vi "Draw Caster Wheel Forward Velocity.vi"(6 "wheel state":T1, 7 "picture info":T3={"picture size"={"Width"=500, "Height"=500}, "pixels per unit"=10.0}, 8 "error in (no error)":errorcluster, 9 "draw wheel options":T2={"global wheel position"={"x"=0.0, "y"=0.0}, "wheel frame angle (rad)"=0.0, "color (black)"=0, "draw wheel state"=FALSE, "draw forward velocity"=FALSE, "velocity scale"=16711680.0, "velocity color (red)"=16711680}, 10 "picture in":picture, 11 "wheel in":refnum<class "NI_Robotics_Wheel.lvclass">) -> (0 "error out":errorcluster, 2 "picture out":picture, 3 "wheel out":refnum<class "NI_Robotics_Wheel.lvclass">)   [LabVIEW 2017, in "NI_Robotics_Steering Picture.lvlib"]
uses:
  <vilib>/robotics/Utilities/Visualization/Steering Visualization/Steering Picture/NI_Robotics_Steering Picture.lvlib
  <vilib>/robotics/Steering/Wheel/NI_Robotics_Wheel.lvclass
  <vilib>/robotics/Utilities/Visualization/Steering Visualization/Steering Picture/Picture Info.ctl
  <vilib>/Utility/miscctls.llb/LVBoundsTypeDef.ctl
  <vilib>/robotics/Utilities/Visualization/Steering Visualization/Steering Picture/Draw Wheel Options.ctl
  <vilib>/robotics/Steering/Wheel/Wheel State.ctl
  <vilib>/Analysis/coordinate.llb/2D Cartesian Coordinate Rotation (Scalar).vi
  <vilib>/Analysis/coordinate.llb/Angle Rotation (scalar).vi
  <vilib>/Analysis/coordinate.llb/2D Cartesian Coordinate Rotation (Array).vi
  <vilib>/robotics/Utilities/Visualization/Steering Visualization/Steering Picture/Global Position to Pixel.vi
  <vilib>/Analysis/coordinate.llb/Wrap Angle (scalar).vi
  <vilib>/picture/picture.llb/Draw Line.vi
  <vilib>/picture/picture.llb/Move Pen.vi
  <vilib>/robotics/Steering/Wheel/Get Caster Wheel Information.vi
  <vilib>/Analysis/NI_AALPro.lvlib
  <vilib>/Analysis/NI_AAL_Angle.lvlib
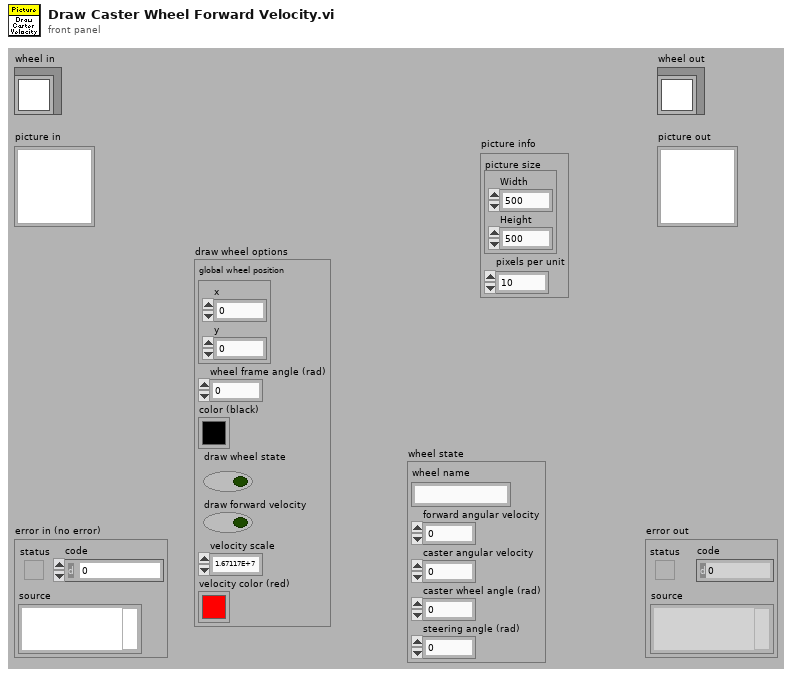
[diagram p1: front panel]
types:
  T1 = typedef "NI_Robotics_Wheel.lvclass/Wheel State.ctl" = cluster{"wheel name":string, "forward angular velocity":dbl, "caster angular velocity":dbl, "caster wheel angle (rad)":dbl, "steering angle (rad)":dbl}
  T2 = typedef "NI_Robotics_Steering Picture.lvlib/Draw Wheel Options.ctl" = cluster{"global wheel position":cluster{"x":dbl, "y":dbl}, "wheel frame angle (rad)":dbl, "color (black)":u32, "draw wheel state":bool, "draw forward velocity":bool, "velocity scale":dbl, "velocity color (red)":u32}
  T3 = typedef "NI_Robotics_Steering Picture.lvlib/Picture Info.ctl" = cluster{"picture size":T4, "pixels per unit":dbl}
  T4 = typedef "LVBoundsTypeDef.ctl" = cluster{"Width":u32, "Height":u32}
  T5 = typedef "NI_Robotics_Caster Wheel.lvclass/Caster Wheel Parameters.ctl" = cluster{"forward offset":dbl, "caster gear ratio":dbl}
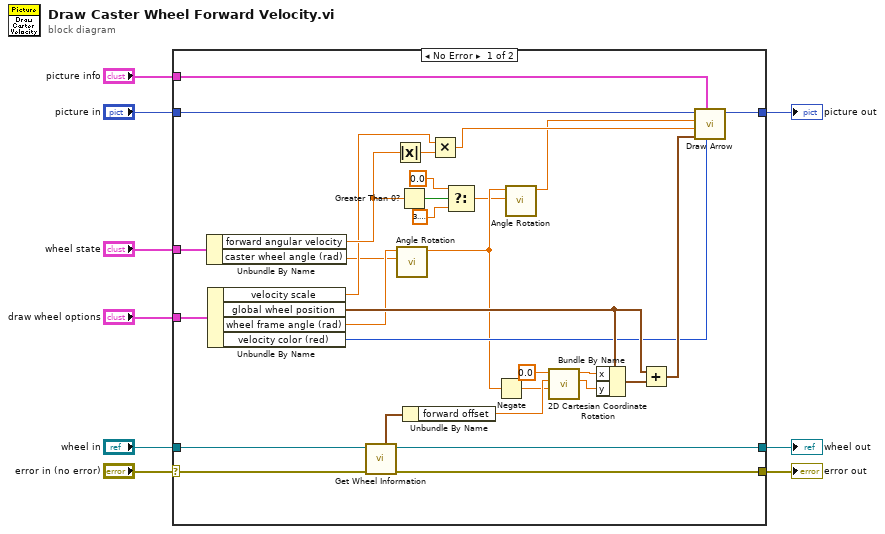
[diagram p0: block diagram]
diagram:
  n1 = case shown="No Error" "error in (no error)" {
    selector: "error in (no error)" -> [w39 w43]
    tunnel: [w38 w43] -> w8
    tunnel: "wheel in" -> [w40 w41]
    tunnel: "picture in" -> [w35 w42]
    tunnel: [w28 w42] -> w5
    tunnel: [w37 w41] -> w4
    tunnel: "picture info" -> [w27 _]
    tunnel: "draw wheel options" -> [w26 _]
    tunnel: "wheel state" -> [w24 _]
    frame No Error {
      n2 = Unbundle By Name(w24) -> ("forward angular velocity"=w17:dbl, "caster wheel angle (rad)"=w13:dbl)
      n3 = Unbundle By Name(w26) -> ("velocity scale"=w15:dbl, "global wheel position"=w25:cluster{"x":dbl, "y":dbl}, "wheel frame angle (rad)"=w14:dbl, "velocity color (red)"=w22:u32)
      n4 = call-poly <vilib>:"Get Wheel Information.vi"("error in (no error)"=w39, "wheel in"=w40) -> ("error out"=w38:errorcluster, "wheel out"=w37:refnum<class "NI_Robotics_Wheel.lvclass">, "caster parameters"=w36:T5)  [unwired: 3 in, 4 out]
      n5 = Absolute Value(x=w17) -> (abs(x)=w21:dbl)
      n6 = call-poly <vilib>:"Angle Rotation.vi"("counterclockwise rotation"=w13, "angle"=w14) -> ("rotated angle"=w12:dbl)  [unwired: 8 in, 1 out]
      n7 = Greater Than 0?(x=w17) -> (x > 0?=w18:bool)
      n8 = Unbundle By Name(w36) -> ("forward offset"=w34:dbl)
      n9 = Multiply(x=w15, y=w21) -> (x*y=w16:dbl)
      n10 = Select(t=0.0, s=w18, f=3.141592653589793) -> (s? t:f=w10:dbl)
      n11 = Negate(x=w12) -> (-x=w32:dbl)
      n12 = call-poly <vilib>:"Angle Rotation.vi"("counterclockwise rotation"=w10, "angle"=w12) -> ("rotated angle"=w11:dbl)  [unwired: 8 in, 1 out]
      n13 = call-poly <vilib>:"2D Cartesian Coordinate Rotation.vi"("theta"=w32, "y"=w34, "x"=0.0) -> ("y out"=w30:dbl, "x out"=w31:dbl)  [unwired: 6 in, 1 out]
      n14 = Bundle By Name(cluster=w25, "x"=w31, "y"=w30) -> (w29:cluster{"x":dbl, "y":dbl})
      n15 = Add(x=w25, y=w29) -> (x+y=w23:cluster{"x":dbl, "y":dbl})
      n16 = call <vilib>:"Draw Arrow.vi"("color"=w22, "picture info"=w27, "global base position"=w23, "length"=w16, "wheel frame angle (rad)"=w11, "picture in"=w35) -> ("picture out"=w28:picture)  [unwired: 5 in]
    }
    frame Error {
    }
  }
  "error out" <- w8
  "wheel out" <- w4
  "picture out" <- w5
